vi "Temp.vi"() -> ()   [LabVIEW 2015]
uses:
  Eagle_RT Globals.vi
panel:
  in  "Lookup Array":fxp<+/-,64,32>[][](array[numeric])
  out "NumericOut":fxp<+/-,16,3>
  in  "NumericIn":fxp<+/-,16,3>
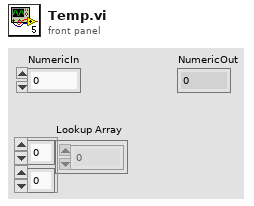
[diagram p1: front panel]
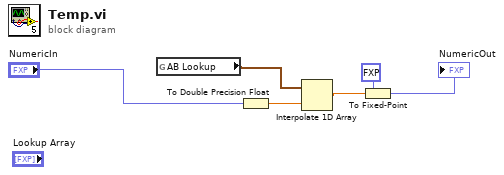
[diagram p0: block diagram]
diagram:
  n1 = global read "Eagle_RT Globals.vi" "AB Lookup"() -> (w6:cluster{"x":dbl, "y":dbl}[])
  n2 = To Double Precision Float(number="NumericIn") -> (double precision float=w5:dbl)
  n3 = Interpolate 1D Array(1:w5, 2:w6) -> (0:w3:dbl)
  n4 = To Fixed-Point(fixed-point type=fxp<+/-,16,3> 0.0, number=w3) -> (fixed-point=→"NumericOut":fxp<+/-,16,3>)
